vi "Start Measurements.vi"(6 "Reply to":refnum<class "Result Reply Msg.lvclass">, 7 "Objects enqueuers":refnum<class "Message Enqueuer.lvclass">[](array[class]), 8 "error in (no error)":errorcluster, 10 "Objects":string[](array[string]), 11 "Measure Controller in":refnum<class "Process Controller.lvclass">) -> (0 "error out":errorcluster, 3 "Measure Controller out":refnum<class "Process Controller.lvclass">)   [LabVIEW 2016, in "Process Controller.lvclass"]
uses:
  Process Controller.lvclass
  C:/github/LabActor/Worker/Worker.lvclass
  Template Module Messages/Result Reply Msg/Result Reply Msg.lvclass
  <vilib>/ActorFramework/Message Enqueuer/Message Enqueuer.lvclass
  Worker/Worker.lvclass/Worker.ctl
  Worker/Worker State.ctl
  Process Controller.lvclass/Process Controller.ctl
  Template Module/Write State.vi
  Worker/Read Cycle period.vi
  Template Module/Read State.vi
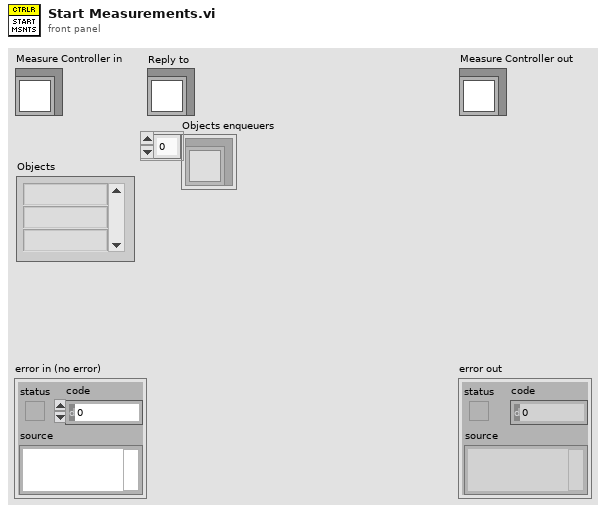
[diagram p1: front panel]
types:
  T1 = typedef "Worker State.ctl" = enum16{"Idle", "Starting", "Working", "Stopping"}
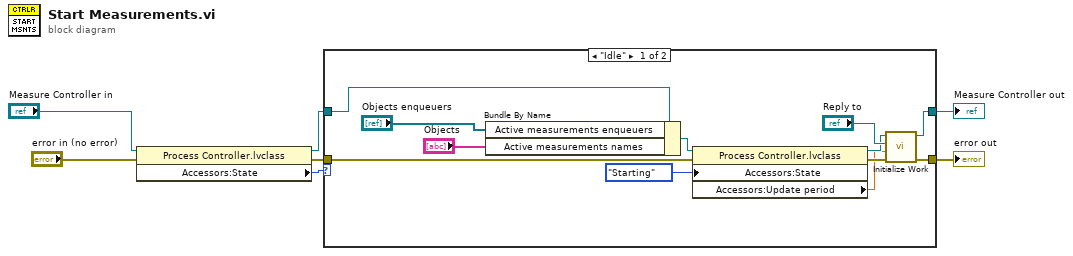
[diagram p0: block diagram]
diagram:
  n1 = property class="Process Controller.lvclass"(reference="Measure Controller in", error in="error in (no error)") -> (reference out=w3:refnum<class "Process Controller.lvclass">, error out=w1:errorcluster, "Accessors:State"=w2:T1)
  n2 = case shown="\"Idle\"" w2 {
    tunnel: [w16 w20] -> w6
    tunnel: [w17 w21] -> w5
    tunnel: w3 -> [w19 w21]
    tunnel: w1 -> [w10 w20]
    frame "Idle" {
      n3 = Bundle By Name(cluster=w19, "Active measurements enqueuers"="Objects enqueuers", "Active measurements names"="Objects") -> (w12:refnum<class "Process Controller.lvclass">)
      n4 = property class="Process Controller.lvclass"(reference=w12, error in=w10, "Accessors:State"=Worker_State."Starting" ("State")) -> (reference out=w11:refnum<class "Process Controller.lvclass">, error out=w13:errorcluster, "Accessors:Update period"=w9:dbl)
      n5 = call-dynamic "Initialize Work.vi"("error in (no error)"=w13, "Update period"=w9, "Reply to"="Reply to", "Measure Controller in"=w11) -> ("error out"=w16:errorcluster, "Measure Controller out"=w17:refnum<class "Process Controller.lvclass">)  [unwired: 6 in]
    }
    frame "Working", Default {
    }
  }
  "error out" <- w6
  "Measure Controller out" <- w5
